vi "Byte Array to U32.vi"(1 "Input Bytes":u8[](array[numeric]) format="%.0x") -> (0 "Output Integers":i32[](array[numeric]))   [LabVIEW 2024]
doc: "Changes unsigned array of bytes into 32 bit signed integers by combining bytes.\nScott Hannahs, NHMFL - FSU, Dec 1997"
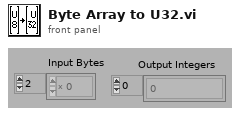
[diagram p1: front panel]
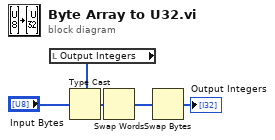
[diagram p0: block diagram]
diagram:
  n1 = local read "Output Integers"() -> (w5:i32[])
  n2 = Type Cast(type=w5, x="Input Bytes") -> (*(type *) &x=w3:i32[])
  n3 = Swap Words(1:w3) -> (0:w2:i32[])
  n4 = Swap Bytes(anything=w2) -> (byte swapped=→"Output Integers":i32[])
